vi "scan2d_close_axis.vi"(8 "error in (no error)":errorcluster, 11 "scan_2d in":refnum<class "scan_2d.lvclass">) -> (0 "error out":errorcluster, 3 "scan_2d out":refnum<class "scan_2d.lvclass">)   [LabVIEW 2015, in "scan_2d.lvclass"]
uses:
  scan_2d.lvclass
  scan_2d.lvclass/scan_2d.ctl
  UI/panel_class/panel.lvclass
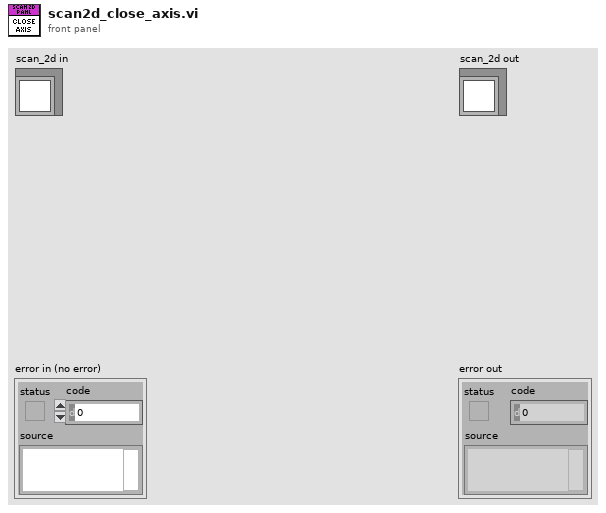
[diagram p1: front panel]
types:
  T1 = typedef "hardware_caller_queue_numbers.ctl" = enum16{"stage1", "stage2", "experiment", "detector"}
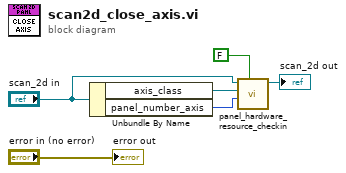
[diagram p0: block diagram]
diagram:
  n1 = Unbundle By Name("scan_2d in") -> ("axis_class"=w5:refnum<class "Stage.lvclass">, "panel_number_axis"=w2:T1)
  n2 = call "panel_hardware_resource_checkin.vi"("Self"=FALSE, "panel_number"=w2, "hardware.lvclass"=w5, "panel in"="scan_2d in") -> ("panel out"=→"scan_2d out":refnum<class "scan_2d.lvclass">)  [unwired: 6 in, 1 out]
  "error out" <- "error in (no error)"
